vi "temp595.vi"() -> ()   [LabVIEW 2010]
panel:
  out "Type K Voltage":dbl
  out "error out":errorcluster
  out "Temperature\nMeasure":T1(ring)
  out "Temperature":dbl
  in  "error in (no error)":errorcluster
  in  "Desired Temperature\nMeasure":T1(ring)
  out "Waveform Chart":dbl(graph)
  in  "Boolean":bool
  in  "stop":bool
  in  "Delay Time (s)":dbl=1.0
  # "Note: Please supply a measured value in volts"
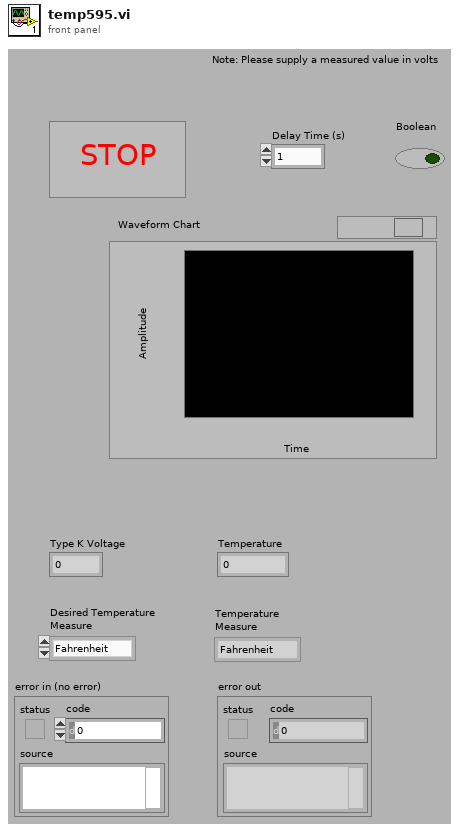
[diagram p1: front panel]
types:
  T1 = enum16{"Fahrenheit", "Celsius", "Kelvin", "Rankine"}
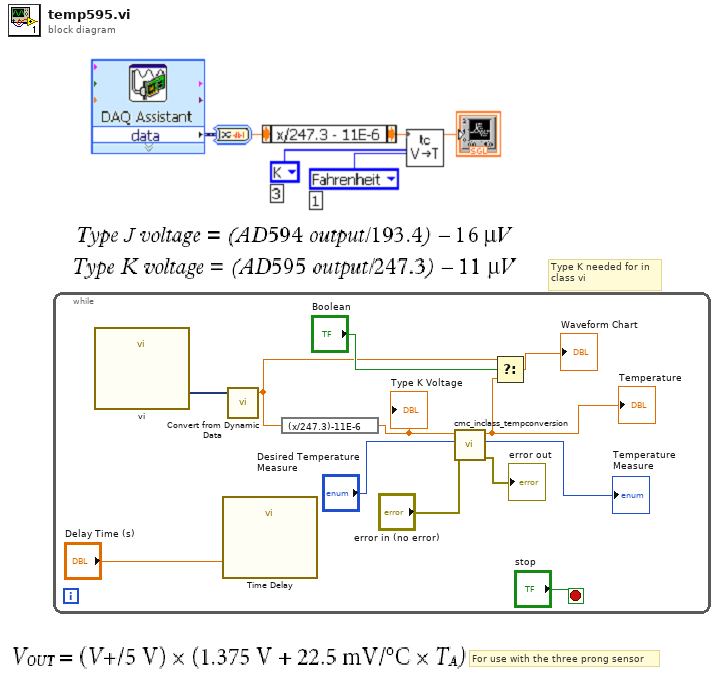
[diagram p0: block diagram]
diagram:
  # "Type K needed for in\nclass vi"
  # "For use with the three prong sensor"
  n1 = while {
    stop <- "stop" stop-if-true
    n2 = call "vi.vi"() -> ("data"=w10:dynamicdata)  [unwired: 17 in, 2 out]
    n3 = call "Time Delay"("Delay Time (s)"="Delay Time (s)") -> ()  [unwired: 10 in, 1 out]
    n4 = call "Convert from Dynamic Data"("Dynamic Data Type"=w10) -> ("Scalar"=w7:dbl)  [unwired: 3 in]
    n5 = expression code="(x/247.3)-11E-6"(w7) -> (w6:dbl)
    "Type K Voltage" <- w6
    n6 = call "cmc_inclass_tempconversion.vi"("error in (no error)"="error in (no error)", "Desired Temperature\nMeasure"="Desired Temperature\nMeasure", "Type K Voltage(V)"=w6) -> ("error out"=→"error out":errorcluster, "Temperature\nMeasure"=→"Temperature\nMeasure":T1, "Temperature"=w1:dbl)  [unwired: 6 in]
    "Temperature" <- w1
    n7 = Select(t=w7, s="Boolean", f=w1) -> (s? t:f=→"Waveform Chart":dbl)
  }
